vi "executeVS_cpp_code.vi"() -> ()   [LabVIEW 2018]
uses:
  scriptsVS/x64/Debug/Dll1.dll
panel:
  in  "arg2":i32=5
  in  "arg1":i32=2
  out "return type":i32
  # ".cpp code called as a library."
  # "="
  # "X"
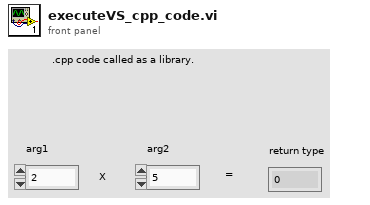
[diagram p1: front panel]
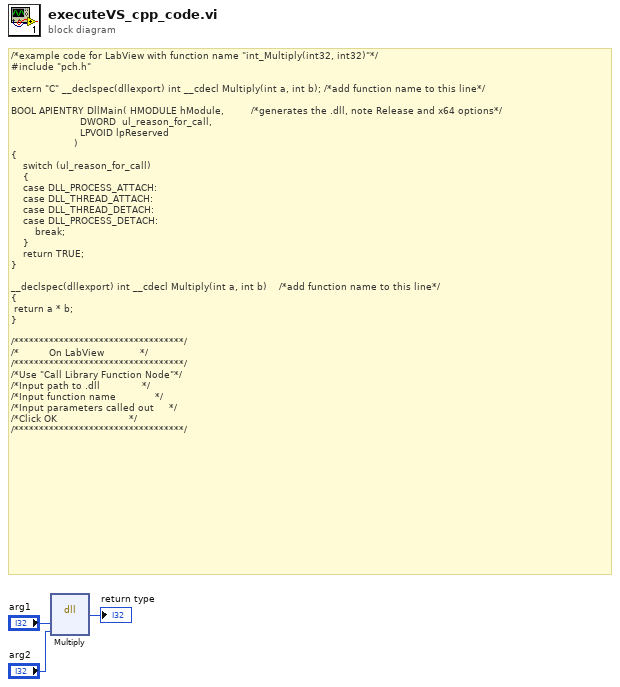
[diagram p0: block diagram]
diagram:
  # "/*example code for LabView with function name \"int_Multiply(int32, int32)\"*/\n#include \"pch.h\"\n\nextern \"C\" __declspec(dllexport) int __cdecl Multiply(int a, int b);\t/*add function name to this line*/\n\nBOOL APIENTRY DllMain( HMODULE hModule,\t\t\t\t\t\t\t\t\t/*generates the .dll, note Release and x64 options*/\n                       DWORD  ul_reason_for_call,\n                       LPVOID lpReserved\n                     )\n{\n    switch (ul_reason_for_call)\n    {\n    case DLL_PROCESS_ATTACH:\n    case DLL_THREAD_ATTACH:\n    case DLL_THREAD_DETACH:\n    case DLL_PROCESS_DETACH:\n        break;\n    }\n    return TRUE;\n}\n\n__declspec(dllexport) int __cdecl Multiply(int a, int b)\t\t\t\t/*add function name to this line*/\n{\n\treturn a * b;\n}\n\n/**********************************/\n/*          On LabView            */\n/**********************************/\n/*Use \"Call Library Function Node\"*/\n/*Input path to .dll              */\n/*Input function name             */\n/*Input parameters called out     */\n/*Click OK                        */\n/**********************************/"
  n1 = dll-call lib="C:/Users/bryan.lee/Documents/GitHub/LabVIEW/learning/LVUexamples/VS/scriptsVS/x64/Debug/Dll1.dll" fn="Multiply"("arg1"="arg1", "arg2"="arg2") -> ("return type"=→"return type":i32)  [unwired: 5 in, 2 out]
